vi "midichannel.set.vi"(8 "error in":errorcluster, 10 "midichannel":u64, 11 "midi in":refnum<class "midi.lvclass">) -> (0 "error out":errorcluster, 3 "midi out":refnum<class "midi.lvclass">)   [LabVIEW 2020, in "midi.lvclass"]
uses:
  midi.lvclass
  midi.lvclass/midi.ctl
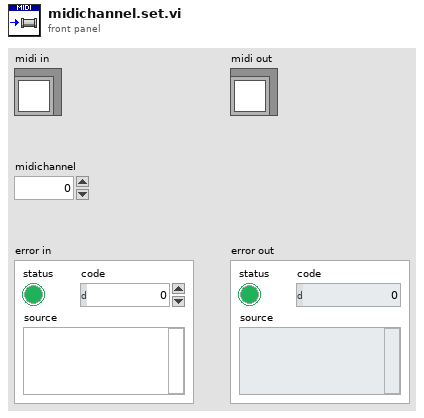
[diagram p1: front panel]
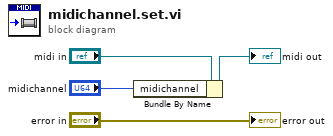
[diagram p0: block diagram]
diagram:
  n1 = Bundle By Name(cluster="midi in", "midichannel"="midichannel") -> (→"midi out":refnum<class "midi.lvclass">)
  "error out" <- "error in"
